vi "Main Control.vi"() -> ()   [LabVIEW 2018]
uses:
  <vilib>/DAQmx/create/channels.llb/DAQmx Create Channel (AI-Voltage-Basic).vi
  cases.ctl
  <vilib>/DAQmx/write.llb/DAQmx Write (Analog DBL 1Chan 1Samp).vi
  cad16ad8-73b1-43df-9668-d44c21423a47.vi
  28c821e5-ae62-4f5b-a0ad-164fd9e515a2.vi
  <vilib>/DAQmx/create/channels.llb/DAQmx Create Channel (AO-Voltage-Basic).vi
  <vilib>/DAQmx/read.llb/DAQmx Read (Analog DBL 1Chan 1Samp).vi
panel:
  in  "retune":T1(ring)
  in  "initialize Button":bool
  out "laser voltage":dbl
  out "reignition voltage":dbl
  out "generator voltage":dbl
  in  "laser":tag
  in  "reigniter":tag
  in  "polarimeter":tag
  in  "RF Generator":tag
  in  "germanium diode":tag
  out "polarimeter threshold":dbl
  out "germanium threshold":dbl
  in  "stop":bool
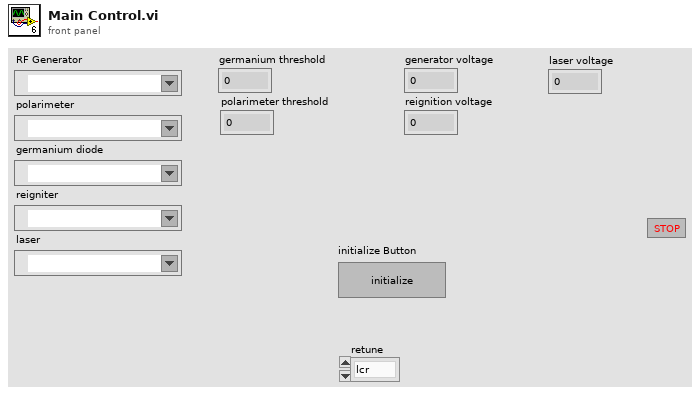
[diagram p1: front panel]
types:
  T1 = enum16{"lcr", "laser", "reigniter", "diodes", "rf generator"}
  T2 = typedef "cases.ctl" = enum16{"set laser voltage", "tune lcr", "tune laser", "quench", "prime", "ignite", "get reignition voltage", "get rf gen ignition voltage", "get ignition threshold", "initialize"}
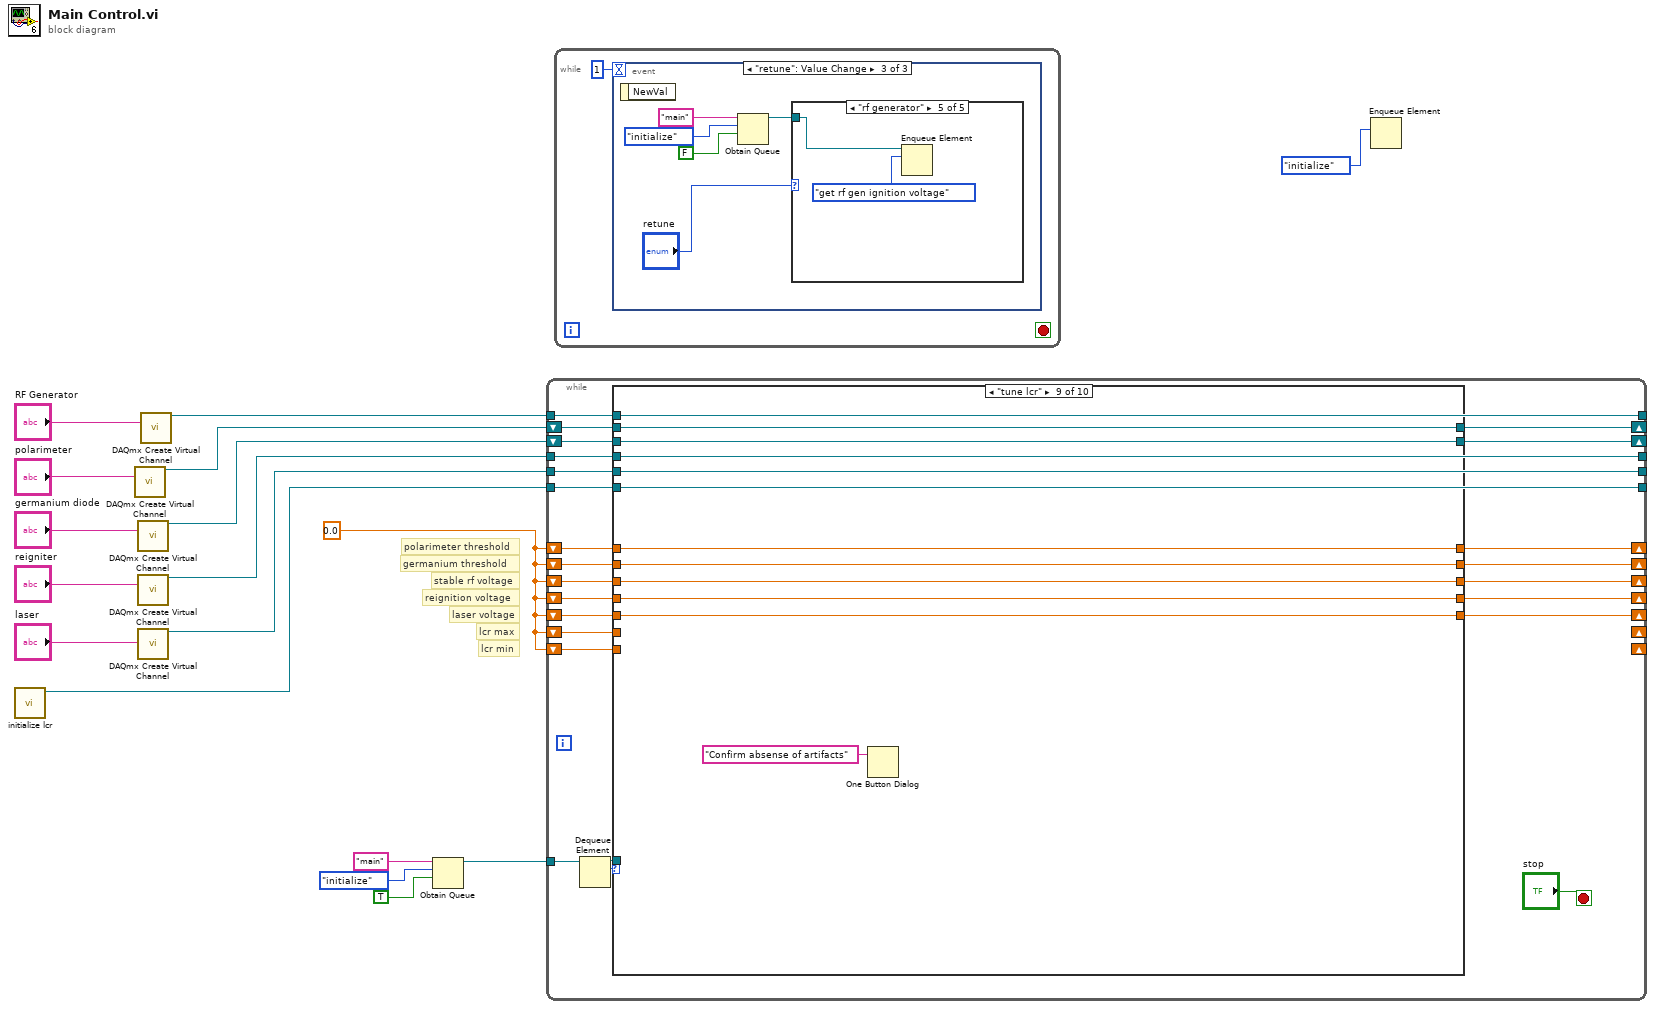
[diagram p0: block diagram]
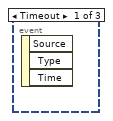
[diagram p2: hidden frame]
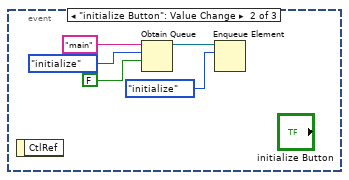
[diagram p3: hidden frame]
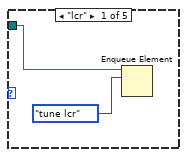
[diagram p4: hidden frame]
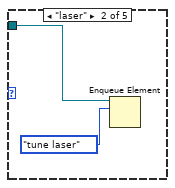
[diagram p5: hidden frame]
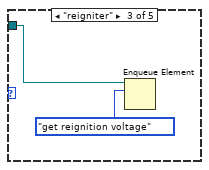
[diagram p6: hidden frame]
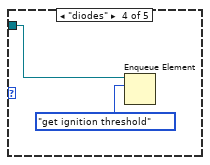
[diagram p7: hidden frame]
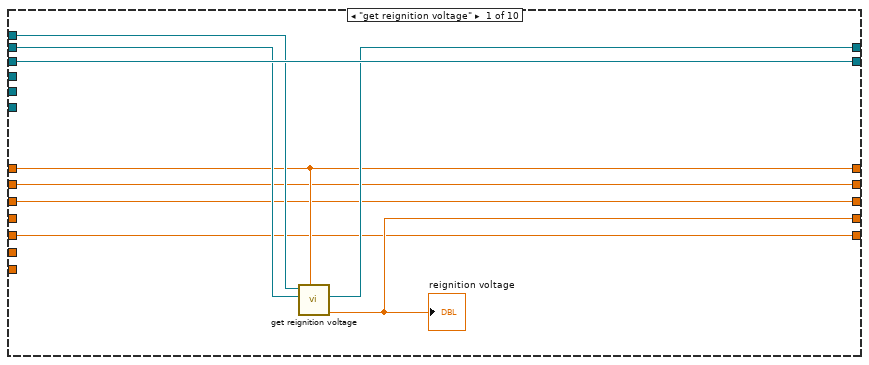
[diagram p8: hidden frame]
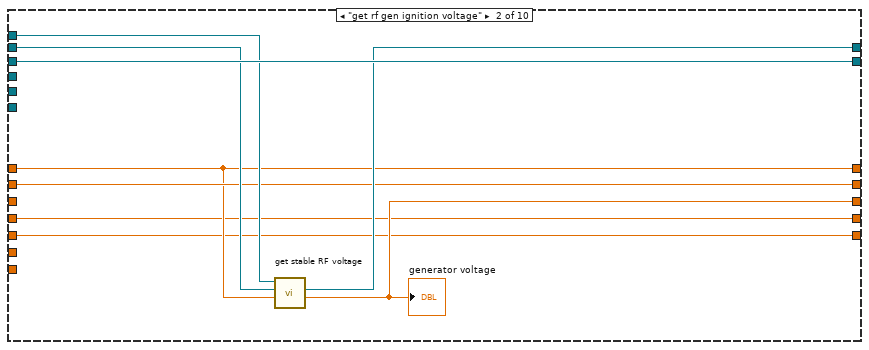
[diagram p9: hidden frame]
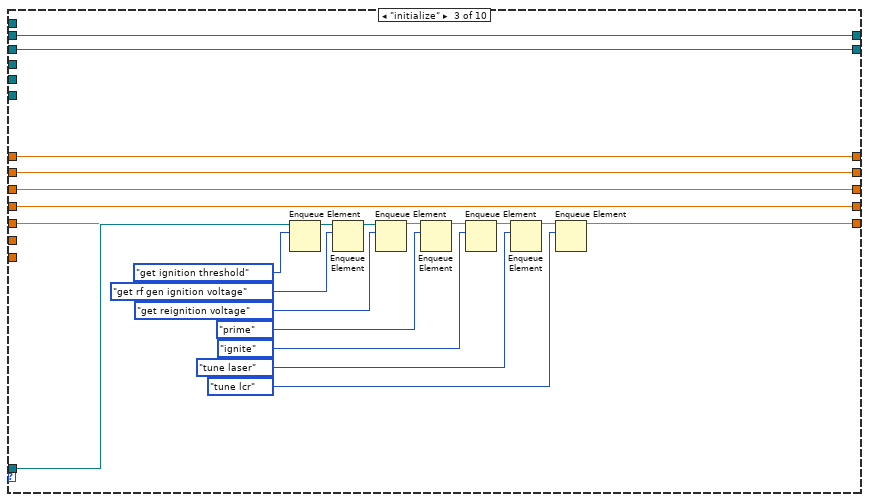
[diagram p10: hidden frame]
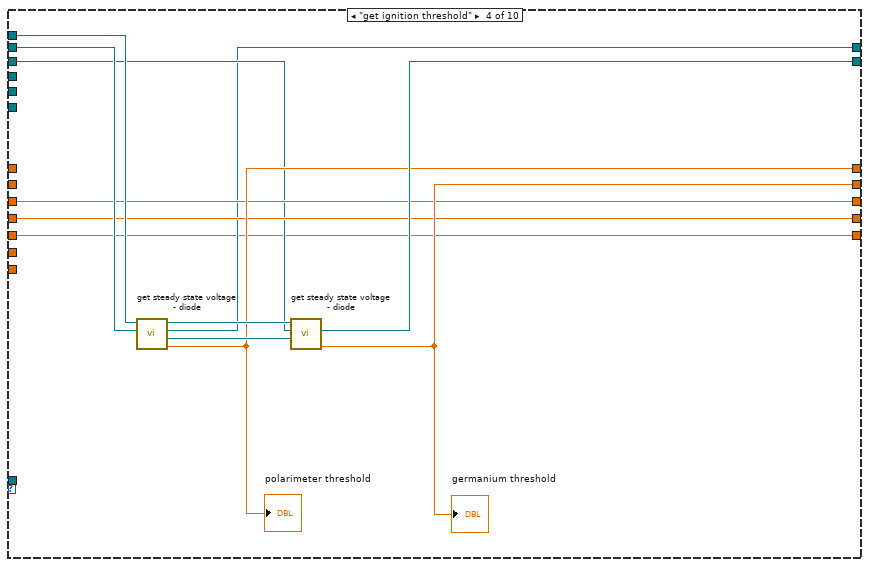
[diagram p11: hidden frame]
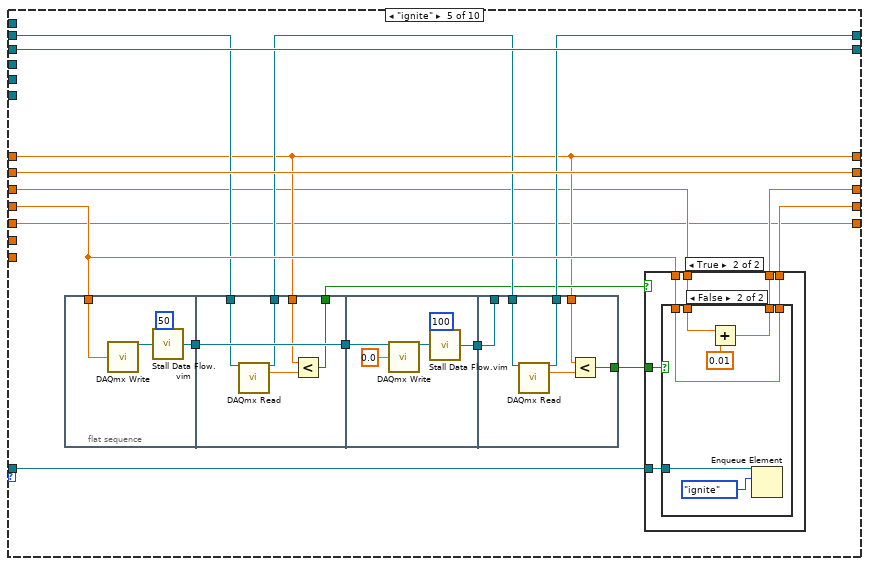
[diagram p12: hidden frame]
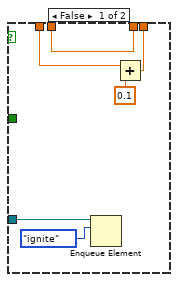
[diagram p13: hidden frame]
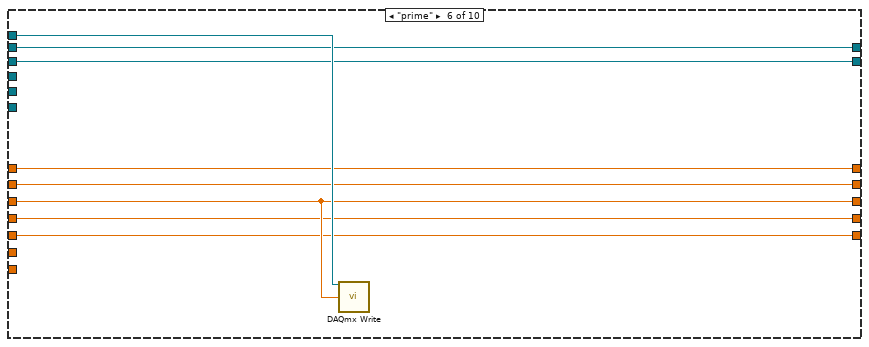
[diagram p15: hidden frame]
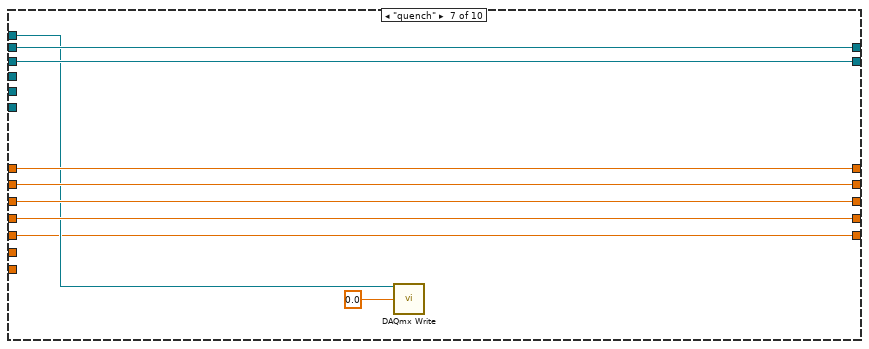
[diagram p16: hidden frame]
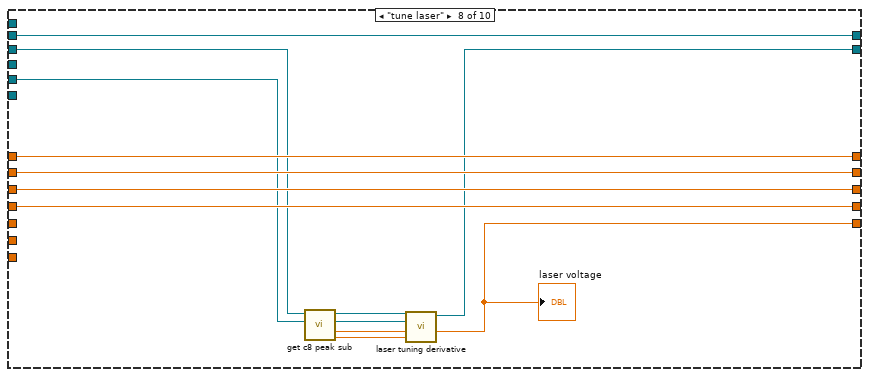
[diagram p17: hidden frame]
diagram:
  w4 = 0.0 ("Output")
  # "lcr max"
  # "lcr min"
  # "laser voltage"
  # "reignition voltage"
  # "germanium threshold"
  # "polarimeter threshold"
  # "stable rf voltage"
  n1 = call "initialize lcr.vi"() -> ("lcr out"=w5:refnum<visa-resource-name>)  [unwired: 11 in]
  n2 = call-poly <vilib>:"DAQmx Create Virtual Channel.vi"("physical channels"="polarimeter") -> ("task out"=w9:refnum<k21>)  [unwired: 13 in, 1 out]
  n3 = call-poly <vilib>:"DAQmx Create Virtual Channel.vi"("physical channels"="germanium diode") -> ("task out"=w8:refnum<k21>)  [unwired: 13 in, 1 out]
  n4 = call-poly <vilib>:"DAQmx Create Virtual Channel.vi"("physical channels"="reigniter") -> ("task out"=w11:refnum<k21>)  [unwired: 13 in, 1 out]
  n5 = call-poly <vilib>:"DAQmx Create Virtual Channel.vi"("physical channels"="laser") -> ("task out"=w6:refnum<k21>)  [unwired: 13 in, 1 out]
  n6 = call-poly <vilib>:"DAQmx Create Virtual Channel.vi"("physical channels"="RF Generator") -> ("task out"=w10:refnum<k21>)  [unwired: 13 in, 1 out]
  n7 = Obtain Queue(name (unnamed)="main", element data type=cases."initialize", create if not found? (T)=TRUE) -> (queue out=w3:refnum<queue>)  [unwired: 2 in, 2 out]
  n8 = while {
    tunnel: w3 -> [w41]
    shift-right: [w35] -> _
    shift-left: w9 -> [w36]
    shift-right: [w34] -> _
    shift-left: w8 -> [w37]
    shift-right: [w33] -> _
    shift-left: w4 -> [w31]
    shift-right: [w32] -> _
    shift-left: w4 -> [w30]
    shift-right: [w29] -> _
    shift-left: w4 -> [w28]
    shift-right: [w27] -> _
    shift-left: w4 -> [w26]
    shift-right: [w24] -> _
    shift-left: w4 -> [w25]
    tunnel: w5 -> [w20]
    tunnel: w10 -> [w23]
    tunnel: w11 -> [w22]
    tunnel: w6 -> [w21]
    tunnel: [w23] -> _
    tunnel: [w22] -> _
    tunnel: [w21] -> _
    tunnel: [w20] -> _
    shift-right: _ -> [_]
    shift-left: w4 -> [w19]
    shift-right: _ -> [_]
    shift-left: w4 -> [w18]
    stop <- "stop" stop-if-true
    n9 = Dequeue Element(queue=w41) -> (queue out=w38:refnum<queue>, element=w40:T2)  [unwired: 2 in, 2 out]
    n10 = case shown="\"tune lcr\"" w40 {
      tunnel: w38 -> [_ _ w80 _ w107 _ _ _ _ _]
      tunnel: w23 -> [w49 w58 _ w92 _ w158 w161 _ _ _]
      tunnel: w37 -> [w50 w59 w73 w83 w109 w156 w166 w170 w187 w194]
      tunnel: w36 -> [w48 w57 w74 w91 w103 w157 w167 w180 w188 w195]
      tunnel: [w47 w56 w74 w82 w101 w157 w167 w180 w188 w195] -> w35
      tunnel: [w50 w59 w73 w88 w109 w156 w166 w174 w187 w194] -> w34
      tunnel: [w46 w54 w72 w87 w97 w155 w163 w179 w186 w193] -> w33
      tunnel: [w44 w55 w71 w86 w108 w154 w162 w178 w185 w192] -> w32
      tunnel: w31 -> [w46 w54 w72 _ w97 w155 w163 w179 w186 w193]
      tunnel: w30 -> [w44 w55 w71 _ w108 w154 w162 w178 w185 w192]
      tunnel: [w43 w53 w70 w85 w94 w153 w164 w177 w184 w191] -> w29
      tunnel: w28 -> [w43 _ w70 w85 w95 w153 w164 w177 w184 w191]
      tunnel: [w45 w52 w69 w84 w98 w152 w165 w176 w183 w190] -> w27
      tunnel: w26 -> [_ w52 w69 w84 w106 w152 w165 w176 w183 w190]
      tunnel: w21 -> [_ _ _ _ _ _ _ w171 _ _]
      tunnel: w25 -> [w42 w51 w68 w81 w93 w151 w159 _ w182 w189]
      tunnel: [w42 w51 w68 w81 w93 w151 w159 w175 w182 w189] -> w24
      tunnel: w20 -> [_ _ _ _ _ _ _ _ _ _]
      tunnel: w22 -> [_ _ _ _ _ _ _ _ _ _]
      tunnel: w19 -> [_ _ _ _ _ _ _ _ _ _]
      tunnel: w18 -> [_ _ _ _ _ _ _ _ _ _]
      frame "get reignition voltage" {
        n11 = call "get reignition voltage.vi"("polarimeter threshold"=w46, "polarimeter task"=w48, "rf generator task"=w49) -> ("Min Reignition Voltage"=w45:dbl, "polarimeter task"=w47:refnum<k21>)  [unwired: 5 in, 2 out]
        "reignition voltage" <- w45
      }
      frame "get rf gen ignition voltage" {
        n12 = call "get stable RF voltage.vi"("diode steady state voltage"=w54, "polarimeter task in"=w57, "rf gen task in"=w58) -> ("stable voltage"=w53:dbl, "polarimeter task out"=w56:refnum<k21>)  [unwired: 6 in, 1 out]
        "generator voltage" <- w53
      }
      frame "initialize" {
        n13 = Enqueue Element(queue=w80, element=cases."get ignition threshold") -> (queue out=w79:refnum<queue>)  [unwired: 2 in, 2 out]
        n14 = Enqueue Element(queue=w79, element=cases."get rf gen ignition voltage") -> (queue out=w78:refnum<queue>)  [unwired: 2 in, 2 out]
        n15 = Enqueue Element(queue=w78, element=cases."get reignition voltage") -> (queue out=w67:refnum<queue>)  [unwired: 2 in, 2 out]
        n16 = Enqueue Element(queue=w67, element=cases."prime") -> (queue out=w66:refnum<queue>)  [unwired: 2 in, 2 out]
        n17 = Enqueue Element(queue=w66, element=cases."ignite") -> (queue out=w65:refnum<queue>)  [unwired: 2 in, 2 out]
        n18 = Enqueue Element(queue=w65, element=cases."tune laser") -> (queue out=w61:refnum<queue>)  [unwired: 2 in, 2 out]
        n19 = Enqueue Element(queue=w61, element=cases."tune lcr") -> ()  [unwired: 2 in, 3 out]
      }
      frame "get ignition threshold" {
        n20 = call "get steady state voltage - diode.vi"("Diode Task In"=w91, "RF Generator Task In"=w92) -> ("Output"=w87:dbl, "reignition task out"=w89:refnum<k21>, "diode task out"=w82:refnum<k21>, "rf generator task out"=w90:refnum<k21>)  [unwired: 6 in]
        "polarimeter threshold" <- w87
        n21 = call "get steady state voltage - diode.vi"("Reignition Task In"=w89, "Diode Task In"=w83, "RF Generator Task In"=w90) -> ("Output"=w86:dbl, "diode task out"=w88:refnum<k21>)  [unwired: 5 in, 2 out]
        "germanium threshold" <- w86
      }
      frame "ignite" {
        n22 = flat-sequence {
          tunnel: w106 -> [w113]
          tunnel: [w110] -> w105
          tunnel: w105 -> [w119]
          tunnel: [w119] -> w104
          tunnel: w103 -> [w118]
          tunnel: [w117] -> w102
          tunnel: w97 -> [w116]
          tunnel: [w114] -> w99
          tunnel: w104 -> [w122]
          tunnel: [w120] -> w100
          tunnel: w102 -> [w130]
          tunnel: [w129] -> w101
          tunnel: [w128] -> _
          tunnel: w100 -> [w128]
          tunnel: w97 -> [w126]
          tunnel: [w125] -> w96
          frame #0 {
            n23 = call-poly <vilib>:"DAQmx Write.vi"("data"=w113) -> ("task out"=w112:refnum<k21>)  [unwired: 12 in, 2 out]
            n24 = call "Stall Data Flow.vim"("value in"=w112, "milliseconds to wait"=u32 50) -> ("value out"=w110:refnum<k21>)  [unwired: 1 out]
          }
          frame #1 {
            n25 = call-poly <vilib>:"DAQmx Read.vi"("task/channels in"=w118) -> ("task out"=w117:refnum<k21>, "data"=w115:dbl)  [unwired: 12 in, 1 out]
            n26 = Less?(x=w116, y=w115) -> (x < y?=w114:bool)
          }
          frame #2 {
            n27 = call-poly <vilib>:"DAQmx Write.vi"("task/channels in"=w122, "data"=0.0) -> ("task out"=w124:refnum<k21>)  [unwired: 11 in, 2 out]
            n28 = call "Stall Data Flow.vim"("value in"=w124, "milliseconds to wait"=u32 100) -> ("value out"=w120:refnum<k21>)  [unwired: 1 out]
          }
          frame #3 {
            n29 = call-poly <vilib>:"DAQmx Read.vi"("task/channels in"=w130) -> ("task out"=w129:refnum<k21>, "data"=w127:dbl)  [unwired: 12 in, 1 out]
            n30 = Less?(x=w126, y=w127) -> (x < y?=w125:bool)
          }
        }
        n31 = case shown="True" w99 {
          tunnel: w107 -> [w136 w137]
          tunnel: w106 -> [w133 w138]
          tunnel: [w132 w142] -> w98
          tunnel: w96 -> [_ w141]
          tunnel: w95 -> [w131 w140]
          tunnel: [w131 w139] -> w94
          frame False {
            n32 = Enqueue Element(queue=w136, element=cases."ignite") -> ()  [unwired: 2 in, 3 out]
            n33 = Add(x=w133, y=0.1) -> (x+y=w132:dbl)
          }
          frame True {
            n34 = case shown="False" w141 {
              tunnel: [w143 w147] -> w142
              tunnel: w140 -> [w144 w149]
              tunnel: [w144 w148] -> w139
              tunnel: w138 -> [w143 w147]
              tunnel: w137 -> [_ w145]
              frame True {
              }
              frame False {
                n35 = Add(x=w149, y=0.01) -> (x+y=w148:dbl)
                n36 = Enqueue Element(queue=w145, element=cases."ignite") -> ()  [unwired: 2 in, 3 out]
              }
            }
          }
        }
      }
      frame "prime" {
        n37 = call-poly <vilib>:"DAQmx Write.vi"("task/channels in"=w158, "data"=w153) -> ()  [unwired: 11 in, 3 out]
      }
      frame "quench" {
        n38 = call-poly <vilib>:"DAQmx Write.vi"("task/channels in"=w161, "data"=0.0) -> ()  [unwired: 11 in, 3 out]
      }
      frame "tune laser" {
        n39 = call "get c8 peak sub.vi"("laser task in"=w171, "germanium task in"=w170) -> ("lower limit"=w168:dbl, "upper limit"=w169:dbl, "laser task out"=w172:refnum<k21>, "germanium task out"=w173:refnum<k21>)  [unwired: 6 in]
        n40 = call "laser tuning derivative.vi"("lower limit"=w168, "upper limit"=w169, "laser task in"=w172, "germanium task in"=w173) -> ("c8 voltage"=w175:dbl, "germanium task out"=w174:refnum<k21>)  [unwired: 5 in, 1 out]
        "laser voltage" <- w175
      }
      frame "tune lcr" {
        n41 = One Button Dialog(message="Confirm absense of artifacts") -> ()  [unwired: 1 in, 1 out]
      }
      frame Default {
      }
    }
  }
  n42 = while {
    stop <- _ stop-if-true
    n43 = event shown="[2] \"retune\": Value Change" {
      selector: _ -> [_ _ _]
      dyn-events: _ -> [_ _ _]
      timeout: 1 -> [_ _ _]
      event Timeout {
        n44 = event-data() -> ()  [unwired: 1 in, 3 out]
      }
      event "initialize Button": Value Change {
        n45 = event-data() -> ()  [unwired: 1 in, 1 out]
        n46 = Obtain Queue(name (unnamed)="main", element data type=cases."initialize", create if not found? (T)=FALSE) -> (queue out=w198:refnum<queue>)  [unwired: 2 in, 2 out]
        n47 = Enqueue Element(queue=w198, element=cases."initialize") -> ()  [unwired: 2 in, 3 out]
      }
      event "retune": Value Change {
        n48 = event-data() -> ()  [unwired: 1 in, 1 out]
        n49 = Obtain Queue(name (unnamed)="main", element data type=cases."initialize", create if not found? (T)=FALSE) -> (queue out=w202:refnum<queue>)  [unwired: 2 in, 2 out]
        n50 = case shown="\"rf generator\"" "retune" {
          tunnel: w202 -> [w207 w209 w211 w213 w215]
          frame "lcr" {
            n51 = Enqueue Element(queue=w207, element=cases."tune lcr") -> ()  [unwired: 2 in, 3 out]
          }
          frame "laser" {
            n52 = Enqueue Element(queue=w209, element=cases."tune laser") -> ()  [unwired: 2 in, 3 out]
          }
          frame "reigniter" {
            n53 = Enqueue Element(queue=w211, element=cases."get reignition voltage") -> ()  [unwired: 2 in, 3 out]
          }
          frame "diodes" {
            n54 = Enqueue Element(queue=w213, element=cases."get ignition threshold") -> ()  [unwired: 2 in, 3 out]
          }
          frame "rf generator" {
            n55 = Enqueue Element(queue=w215, element=cases."get rf gen ignition voltage") -> ()  [unwired: 2 in, 3 out]
          }
        }
      }
    }
  }
  n56 = Enqueue Element(element=cases."initialize") -> ()  [unwired: 3 in, 3 out]
